vi "Max Current.vi"() -> (0 "Currents By Channel":dbl[](array[numeric]), 1 "Current":dbl format="%#_13g", 2 "Max Amps":dbl=500.0 format="%#_13g")   [LabVIEW 2015]
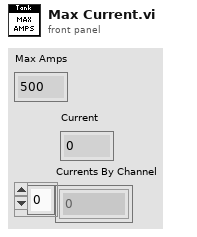
[diagram p1: front panel]
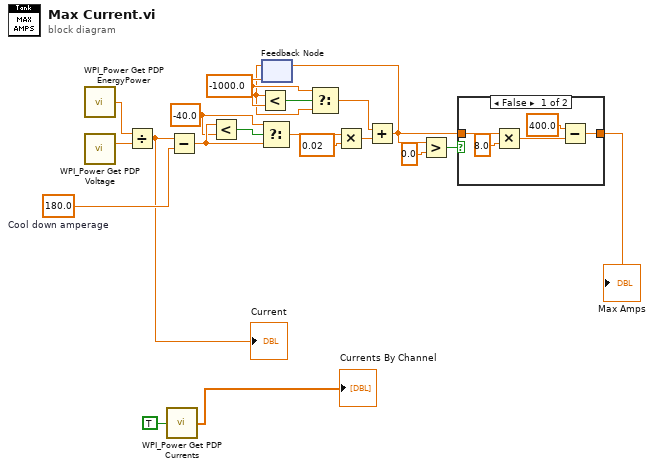
[diagram p0: block diagram]
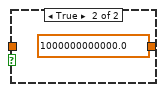
[diagram p2: hidden frame]
diagram:
  w15 = -40.0 ("y")
  w18 = 180.0  # Cool down amperage
  w13 = -1000.0
  n1 = call <vilib>:"WPI_Power Get PDP EnergyPower.vi"() -> ("Power (W)"=w20:dbl)  [unwired: 13 in, 2 out]
  n2 = call <vilib>:"WPI_Power Get PDP Voltage.vi"() -> ("voltage (V)"=w19:dbl)  [unwired: 14 in, 1 out]
  n3 = Divide(x=w20, y=w19) -> (x/y=w3:dbl)
  "Current" <- w3
  n4 = call <vilib>:"WPI_Power Get PDP Currents.vi"("Tare Currents?"=TRUE) -> ("all currents (A)"=→"Currents By Channel":dbl[])  [unwired: 12 in, 2 out]
  n5 = Subtract(x=w3, y=w18) -> (x-y=w16:dbl)
  n6 = Less?(x=w16, y=w15) -> (x < y?=w17:bool)
  n7 = Select(t=w15, s=w17, f=w16) -> (s? t:f=w9:dbl)
  n8 = feedback #1(w13) -> (w12:dbl)
  n9 = Less?(x=w12, y=w13) -> (x < y?=w14:bool)
  n10 = Select(t=w13, s=w14, f=w12) -> (s? t:f=w11:dbl)
  n11 = Multiply(x=w9, y=0.02) -> (x*y=w8:dbl)
  n12 = Add(x=w11, y=w8) -> (x+y=w5:dbl)
  n13 = feedback-in #1(w5) -> ()
  n14 = Greater?(x=w5, y=0.0) -> (0:w6:bool)
  n15 = case shown="False" w6 {
    tunnel: w5 -> [w23 _]
    tunnel: [w21 1000000000000.0] -> w4
    frame False {
      n16 = Multiply(x=w23, y=8.0) -> (x*y=w22:dbl)
      n17 = Subtract(x=400.0, y=w22) -> (x-y=w21:dbl)
    }
    frame True {
    }
  }
  "Max Amps" <- w4
